vi "beep by type.vi"(8 "error in (no error)":errorcluster, 9 "use system alert? (T)":bool, 11 "Type":enum16{"Pass", "Fail"}(ring)=enum."Fail") -> (0 "error out":errorcluster)   [LabVIEW 2013]
panel:
  in  "Type Sound Data":u32[][](array[numeric])=[[1000, 100], [700, 750]]
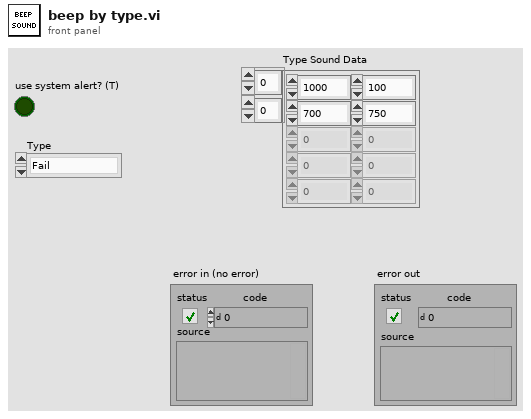
[diagram p1: front panel]
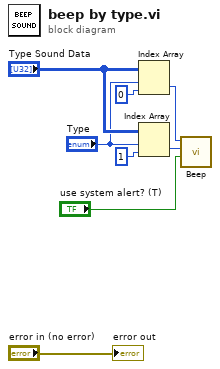
[diagram p0: block diagram]
diagram:
  n1 = Index Array(array="Type Sound Data", index (row)="Type", index (col)=0 ("disabled index (col)")) -> (element=w5:u32)
  n2 = Index Array(array="Type Sound Data", index (row)="Type", index (col)=1 ("disabled index (col)")) -> (element=w2:u32)
  n3 = call <vilib>:"Beep.vi"("use system alert? (T)"="use system alert? (T)", "duration (msec)"=w2, "frequency (Hz)"=w5) -> ()  [unwired: 9 in]
  "error out" <- "error in (no error)"
